vi "Player Info.vi"(11 "Scout in":refnum<class "Scout.lvclass">) -> (1 "Victory Speech":string, 2 "Name":string, 3 "Scout out":refnum<class "Scout.lvclass">)   [LabVIEW 2015, in "Scout.lvclass"]
uses:
  Scout.lvclass
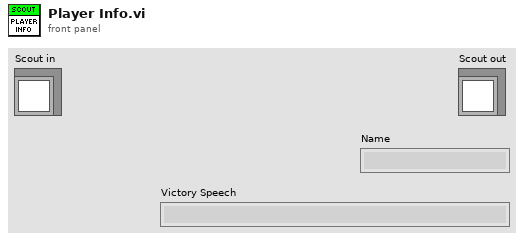
[diagram p1: front panel]
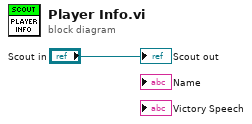
[diagram p0: block diagram]
diagram:
  "Scout out" <- "Scout in"
